vi "SeverityFromString.vi"(6 "Context":string, 8 "error in (no error)":errorcluster, 11 "SeverityString":string) -> (0 "error out":errorcluster, 3 "Severity":T1)   [LabVIEW 2026, in "Lumberjack.lvlib"]
uses:
  Lumberjack.lvlib
  TypeDefs/Severity.ctl
  <vilib>/Utility/error.llb/Trim Whitespace (string).vi
  <vilib>/Utility/error.llb/Trim Whitespace One-Sided.vi
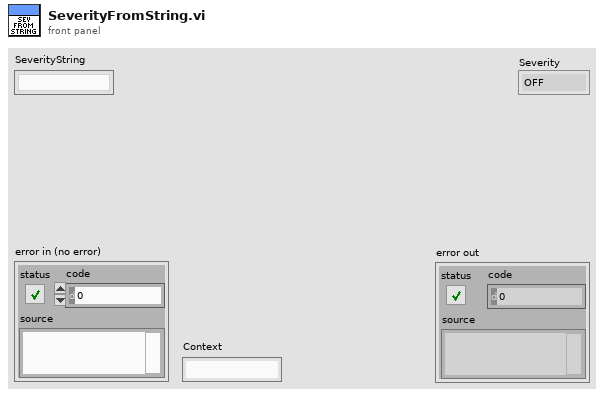
[diagram p1: front panel]
types:
  T1 = typedef "Lumberjack.lvlib/Severity.ctl" = enum16{"OFF", "FATAL", "ERROR", "WARN", "INFO", "DEBUG", "TRACE", "ALL"}
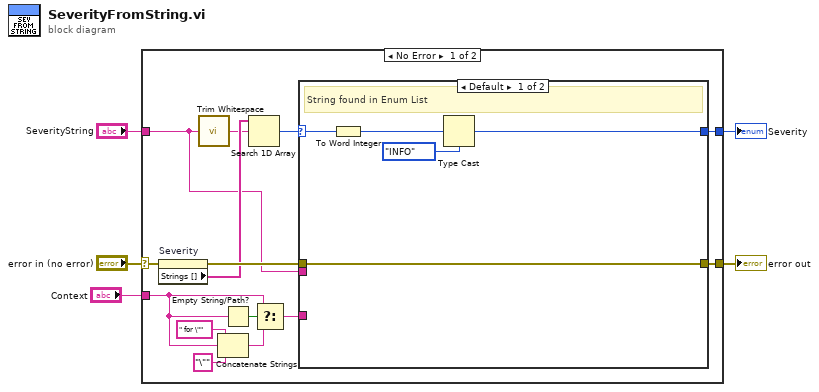
[diagram p0: block diagram]
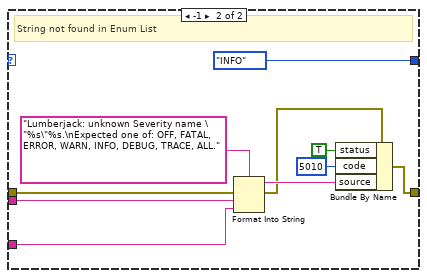
[diagram p2: hidden frame]
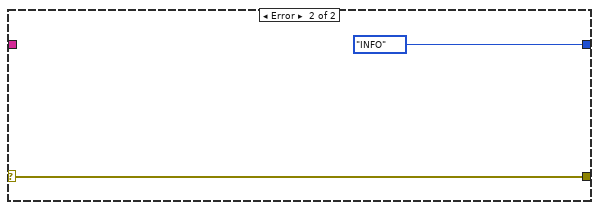
[diagram p3: hidden frame]
diagram:
  n1 = case shown="No Error" "error in (no error)" {
    selector: "error in (no error)" -> [w19 w36]
    tunnel: [w17 w36] -> w5
    tunnel: "SeverityString" -> [w6 _]
    tunnel: [w16 Severity."INFO" ("Severity")] -> w2
    tunnel: "Context" -> [w9 _]
    frame No Error {
      n2 = property on="Severity" class="Enum (strict)"(error in=w19) -> (error out=w18:errorcluster, "Strings []"=w15:string[])  [unwired: 1 in, 1 out]
      n3 = call-poly <vilib>:"Trim Whitespace.vi"("string"=w6) -> ("trimmed string"=w7:string)  [unwired: 1 in]
      n4 = Concatenate Strings(" for \"" ("string"), w9, "\"" ("string")) -> (w11:string)
      n5 = Empty String/Path?(string/path=w9) -> (empty?=w10:bool)
      n6 = Search 1D Array(1D array=w15, element=w7) -> (index of element=w14:i32)  [unwired: 1 in]
      n7 = Select(t=w9, s=w10, f=w11) -> (s? t:f=w8:string)
      n8 = case shown="Default" w14 {
        selector: w14 -> [w21 _]
        tunnel: w18 -> [w24 w29]
        tunnel: [w24 w34] -> w17
        tunnel: [w23 Severity."INFO" ("Severity")] -> w16
        tunnel: w8 -> [_ w25]
        tunnel: w6 -> [_ w26]
        frame Default {
          # "String found in Enum List"
          n9 = To Word Integer(number=w21) -> (16bit integer=w20:i16)
          n10 = Type Cast(type=Severity."INFO" ("Severity"), x=w20) -> (*(type *) &x=w23:T1)
        }
        frame -1 {
          # "String not found in Enum List"
          n11 = Format Into String(format string="Lumberjack: unknown Severity name \"%s\"%s.\nExpected one of: OFF, FATAL, ERROR, WARN, INFO, DEBUG, TRACE, ALL." ("source"), error in=w29, w26, w25) -> (resulting string=w28:string, error out=w27:errorcluster)  [unwired: 1 in]
          n12 = Bundle By Name(cluster=w27, "status"=TRUE, "code"=5010, "source"=w28) -> (w34:errorcluster)
        }
      }
    }
    frame Error {
    }
  }
  "Severity" <- w2
  "error out" <- w5
